vi "Lock-in Globles Multiple Inputs and Outputs.vi"() -> ()   [LabVIEW 2011, in "Lock-In Variable Channels_2.lvclass"]
uses:
  Variable Channel O.O.P/Lock-In Variable Channels_2.lvclass
panel:
  in  "Take Curve":bool
  out "Busy":bool
  in  "Sampling information":cluster{"Fs":dbl, "#s":dbl}[](array[cluster])=[{"Fs"=100000.0, "#s"=200000.0}, {"Fs"=100000.0, "#s"=200000.0}]
  out "Reset Lockin":bool
  in  "OSC Configuration":T1(array[cluster])=[[{"Signal Type"=enum."Sine Wave", "DC"=0.0003, "Amplitude"=0.0005, "frequency"=1.3459999999999999, "Phase"=0.0}, {"Signal Type"=enum."Sine Wave", "DC"=0.0, "Amplitude"=0.0, "frequency"=1.346, "Phase"=0.0}, {"Signal Type"=enum."Sine Wave", "DC"=0.0, "Amplitude"=0.0, "frequency"=1.346, "Phase"=0.0}, {"Signal Type"=enum."Sine Wave", "DC"=0.0, "Amplitude"=0.0, "frequency"=1.346, "Phase"=0.0}]] {"frequency" step=0.001 format="%.3p"; "Amplitude" format="%0.2p"; "DC" min=-0.99 max=0.99 format="%.2p"}
  out "timestamp":timestamp
  in  "Multiplication factor":dbl=1.0
  out "Stop Read current vs T":bool
  out "Input signal":dbl[][](graph)
  out "Stop Lockin":bool
  out "Results":dbl[][](array[numeric])=[[1.4839408729757508e-11, -1.900879392885926e-12, 1.4960661546706472e-11, -7.299647829275913], [1.7200124080450918e-16, -5.0346392409039706e-17, 1.7921826376487348e-16, -16.315253344298398], [1.1117395670783847e-11, -2.59351111233741e-11, 2.8217485279211652e-11, -66.79702725745167], [-3.930657765785384e-11, 1.8195590831737717e-12, 3.934867014817724e-11, 177.3495865094821]]
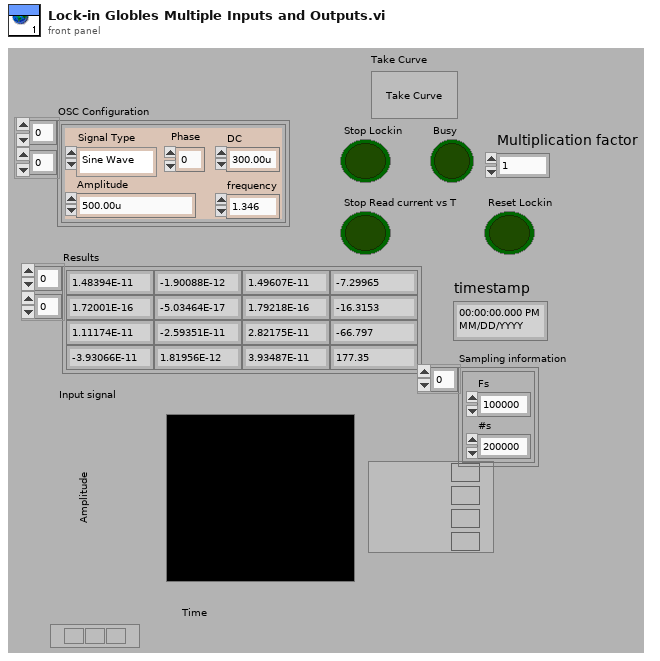
[diagram p1: front panel]
types:
  T1 = cluster{"Signal Type":enum16{"Sine Wave", "Triangle Wave", "Square Wave", "Sawtooth Wave"}, "DC":dbl, "Amplitude":dbl, "frequency":dbl, "Phase":dbl}[][]
diagram:
